vi "Flatten Value.vi"(8 "error in":errorcluster, 11 "2D Flt In":refnum<class "2D Flt.lvclass">) -> (0 "error out":errorcluster, 1 "Value":string, 3 "2D Flt Out":refnum<class "2D Flt.lvclass">)   [LabVIEW 2020, in "NI_VIAnCFGDataStructure.lvlib" / "2D Flt.lvclass"]
doc: "Dynamic dispatch interface for flattening Tree Data classes to string."
uses:
  <vilib>/addons/analyzer/VIAnCFGDataStructure/Data Types/2D Flt/2D Flt.lvclass
  <vilib>/addons/analyzer/VIAnCFGDataStructure/Data Types/2D Flt/2D Flt.lvclass/2D Flt.ctl
  <vilib>/addons/analyzer/VIAnCFGDataStructure/Tree Manager/Tree.lvclass
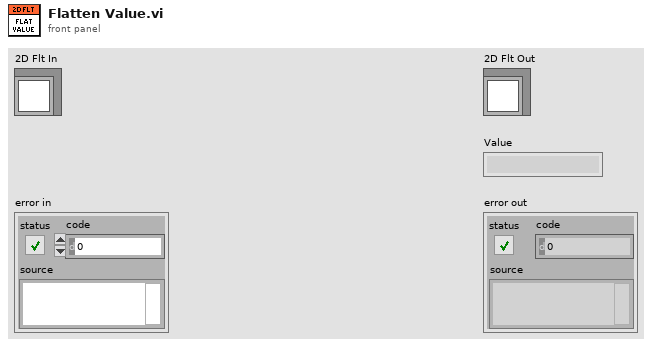
[diagram p1: front panel]
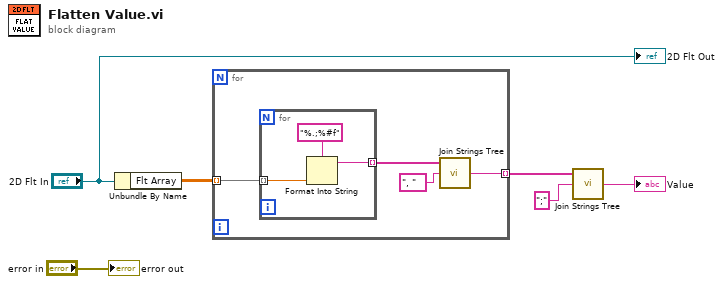
[diagram p0: block diagram]
diagram:
  n1 = Unbundle By Name("2D Flt In") -> ("Flt Array"=w5:dbl[][])
  n2 = for {
    tunnel: w5 -> [w10] mode=indexing
    tunnel: [w7] -> w6 mode=indexing
    n3 = for {
      tunnel: w10 -> [w13] mode=indexing
      tunnel: [w12] -> w9 mode=indexing
      n4 = Format Into String(format string="%.;%#f" ("initial string"), w13) -> (resulting string=w12:string)  [unwired: 2 in, 1 out]
    }
    n5 = call <vilib>:"Join Strings Tree.vi"("Separator (,)"=", ", "Strings In"=w9) -> ("String"=w7:string)  [unwired: 1 in]
  }
  n6 = call <vilib>:"Join Strings Tree.vi"("Separator (,)"=";", "Strings In"=w6) -> ("String"=→"Value":string)  [unwired: 1 in]
  "2D Flt Out" <- "2D Flt In"
  "error out" <- "error in"
